vi "signal traffic.vi"() -> ()   [LabVIEW 2026]
panel:
  in  "stop":bool
  out "green 3":bool
  out "yellow":bool
  out "red 3":bool
  out "green":bool
  out "yellow 2":bool
  out "red 2":bool
  out "green":bool
  out "yellow":bool
  out "red":bool
  out "coerced(x)":dbl
  out "2 frame":dbl
  out "1 frame":dbl
  out "greater than 28":bool
  out "3 frame":dbl
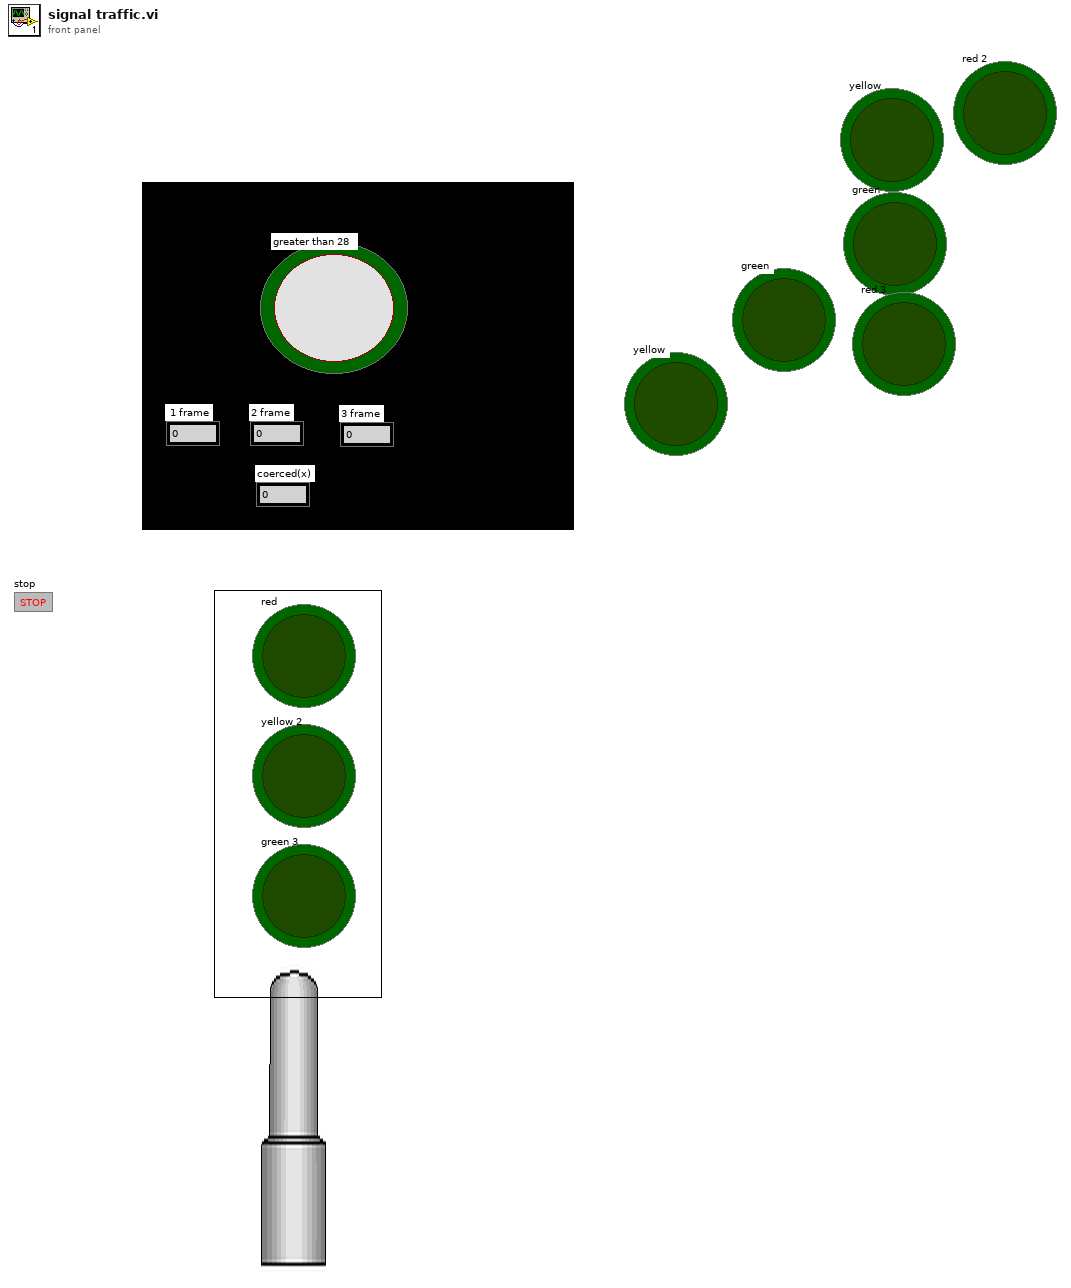
[diagram p1: front panel]
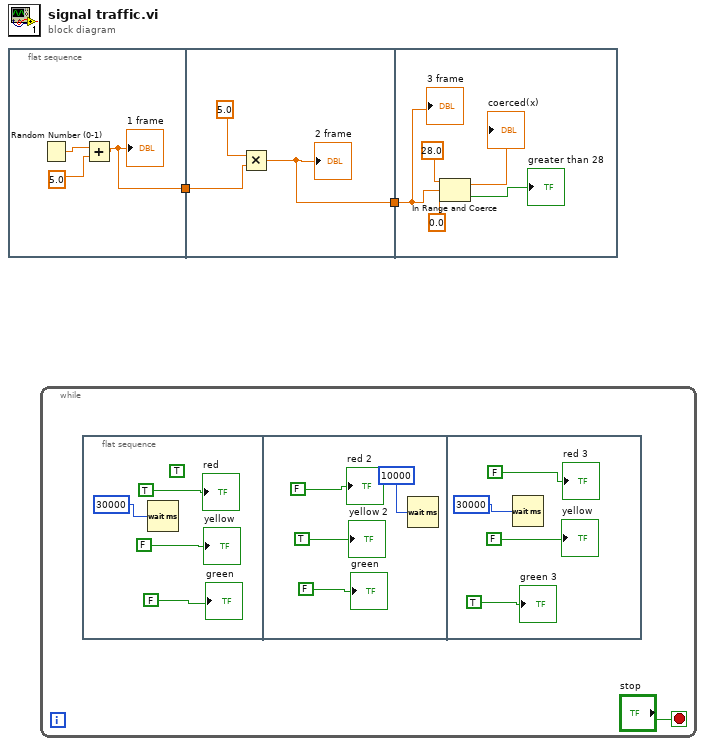
[diagram p0: block diagram]
diagram:
  n1 = flat-sequence {
    tunnel: [w3] -> w2
    tunnel: w2 -> [w8]
    tunnel: [w6] -> w1
    tunnel: w1 -> [w11]
    frame #0 {
      n2 = Random Number (0-1)() -> (number: 0 to 1=w5:dbl)
      n3 = Add(x=w5, y=5.0) -> (x+y=w3:dbl)
      "1 frame" <- w3
    }
    frame #1 {
      n4 = Multiply(x=5.0, y=w8) -> (x*y=w6:dbl)
      "2 frame" <- w6
    }
    frame #2 {
      n5 = In Range and Coerce(upper limit=28.0, x=w11, lower limit=0.0) -> (coerced(x)=→"coerced(x)":dbl, In Range?=→"greater than 28":bool)
      "3 frame" <- w11
    }
  }
  n6 = while {
    stop <- "stop" stop-if-true
    n7 = flat-sequence {
      frame #0 {
        (unwired) TRUE
        n8 = Wait (ms)(milliseconds to wait=u32 30000) -> ()  [unwired: 1 out]
        "red" <- TRUE
        "yellow" <- FALSE
        "green" <- FALSE
      }
      frame #1 {
        n9 = Wait (ms)(milliseconds to wait=u32 10000) -> ()  [unwired: 1 out]
        "green" <- FALSE
        "yellow 2" <- TRUE
        "red 2" <- FALSE
      }
      frame #2 {
        n10 = Wait (ms)(milliseconds to wait=u32 30000) -> ()  [unwired: 1 out]
        "yellow" <- FALSE
        "green 3" <- TRUE
        "red 3" <- FALSE
      }
    }
  }
